vi "Pockels Cal-Succes complet msg.vi"(8 "error in (no error)":errorcluster, 11 "Updated existing file?":bool) -> (0 "error out":errorcluster)   [LabVIEW 2020]
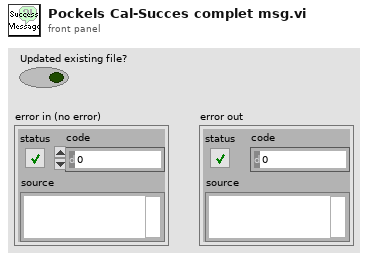
[diagram p1: front panel]
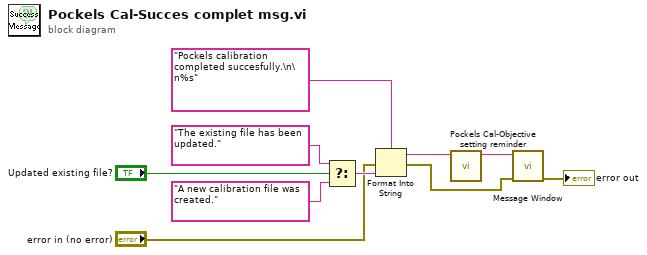
[diagram p0: block diagram]
diagram:
  n1 = Select(t="The existing file has been updated." ("Message string"), s="Updated existing file?", f="A new calibration file was created." ("Message string")) -> (s? t:f=w9:string)
  n2 = Format Into String(format string="Pockels calibration completed succesfully.\n\n%s" ("Message string"), error in="error in (no error)", w9) -> (resulting string=w3:string, error out=w1:errorcluster)  [unwired: 1 in]
  n3 = call "Pockels Cal-Objective setting reminder.vi"("Message in"=w3) -> ("Message"=w2:string)  [unwired: 10 in]
  n4 = call "Message Window.vi"("error in (no error)"=w1, "Message string"=w2) -> ("error out (no error)"=→"error out":errorcluster)  [unwired: 9 in]
